vi "BasicDigitizerAcquire.vi"() -> ()   [LabVIEW 2014]
uses:
  Program Files (x86)/CAEN/Comm/labview/CAENComm.lvlib
panel:
  out "VernierTopHalves":i32[](array[numeric])
  out "QDC":u32[](array[numeric]) format="%.0x"
  in  "QDC module Base Address":u32 format="%.0x"
  in  "# of events before transfer":u16=1 min=1 max=32
  out "error out 2":errorcluster
  in  "# Rpts Vernier Cal":i32=100
  out "Min Ch0":u16
  out "max Ch0":u16
  out "Min Ch2":u16
  out "max Ch2":u16
  out "max Ch1":u16
  out "Min Ch1":u16
  out "Min Ch3":u16
  out "max Ch3":u16
  out "Verniers":u16[][](graph)
  out "End Idx":u16
  out "TRIG_REC":u8
  in  "MBLT?":bool
  out "Mean Time (secs)":dbl
  out "This Time (secs)":dbl
  out "RAW Wfm Plot":u16[](graph)
  in  "stop":bool
  in  "Software Trig?":bool
  in  "VME Base Address":u32=4026859520 format="%.0x"
  out "error out":errorcluster
  out "Wfm Plot":u16[][](graph)
  out "Ch1":u16[](array[numeric])
  out "Ch3":u16[](array[numeric])
  out "Ch0":u16[](array[numeric])
  out "Ch2":u16[](array[numeric])
  out "Channel Data (interleaved)":u32[](array[numeric])
  out "1st Sample, Verniers, and BL Reset":u16[](array[numeric])
  in  "# Samples after Trig":u16
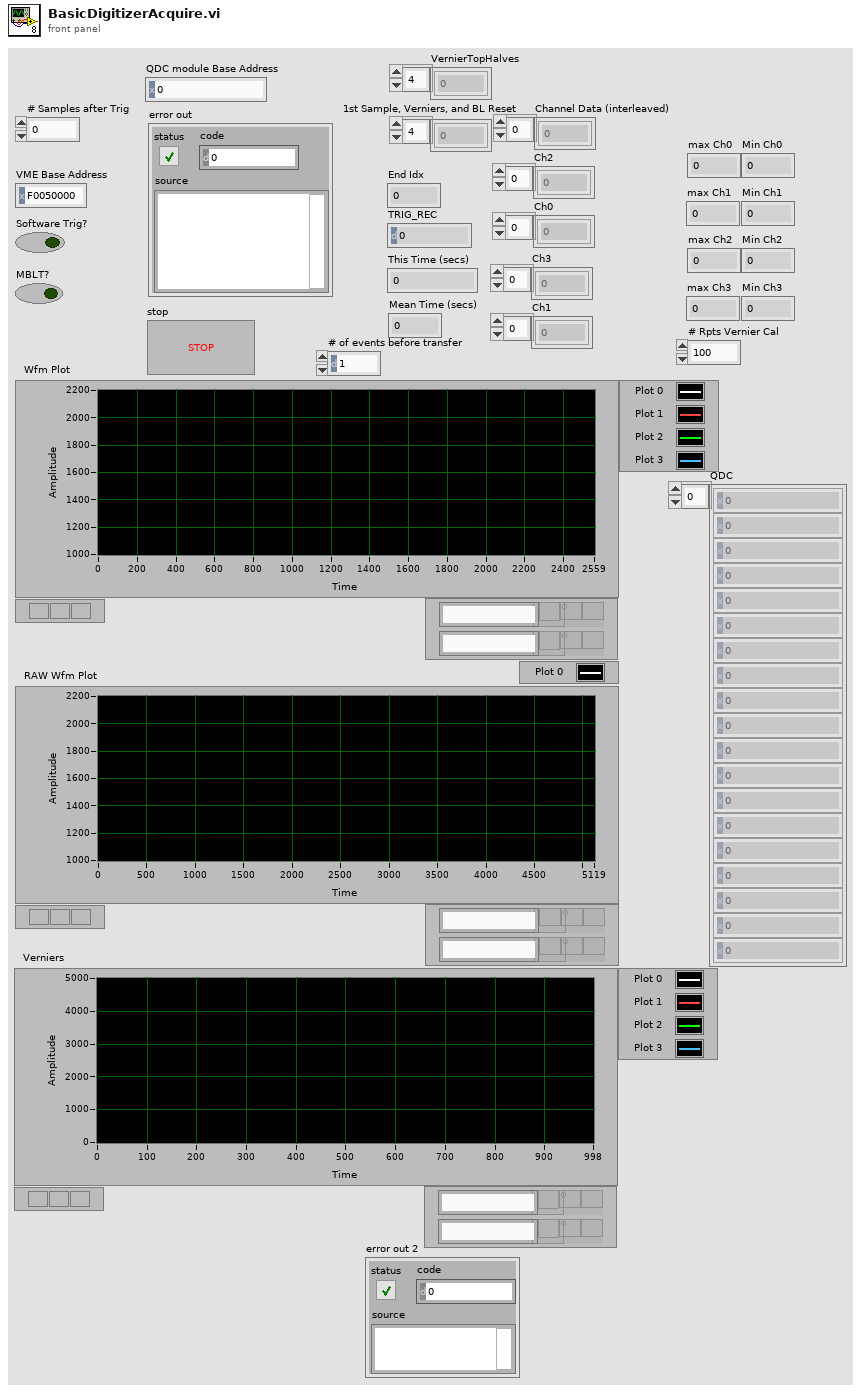
[diagram p1: front panel]
types:
  T1 = enum16{"Configure", "Initialise", "Run", "Close"}
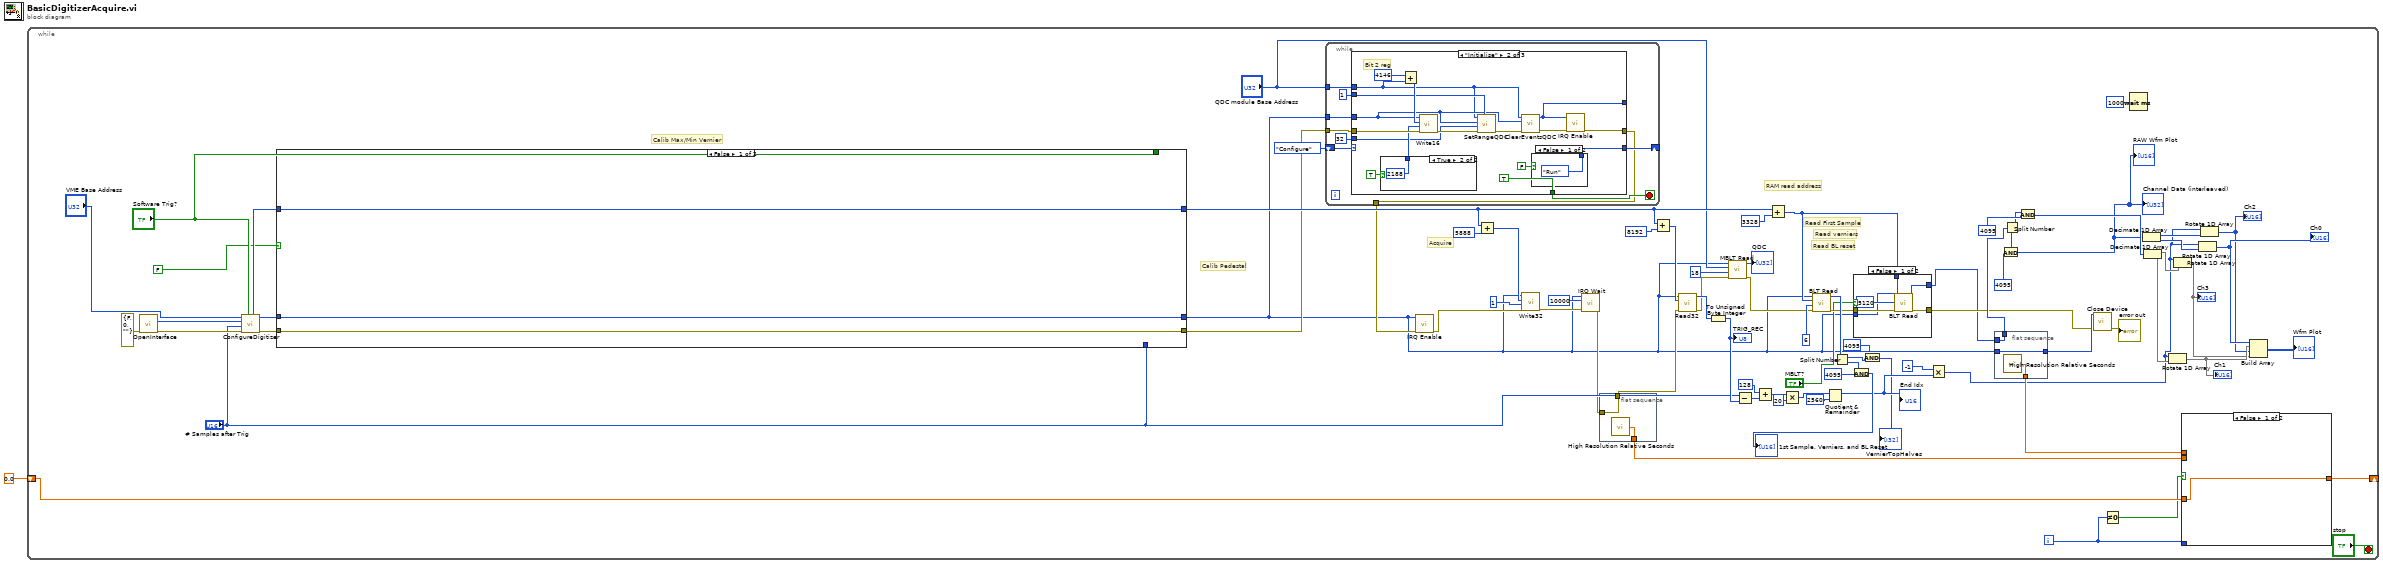
[diagram p0: block diagram]
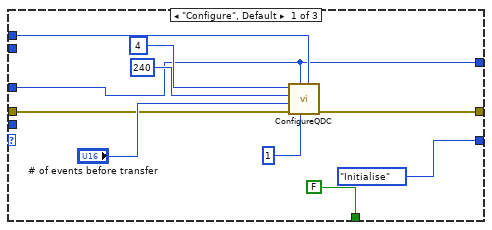
[diagram p2: hidden frame]
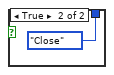
[diagram p3: hidden frame]
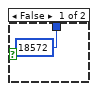
[diagram p4: hidden frame]
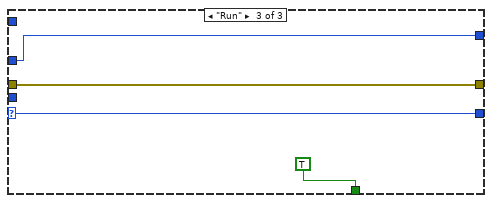
[diagram p5: hidden frame]
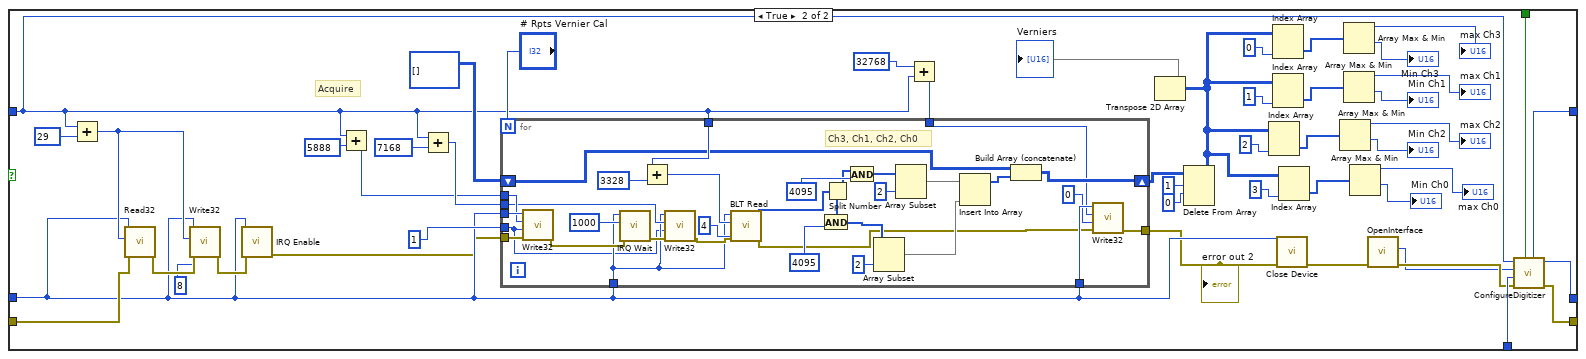
[diagram p6: hidden frame]
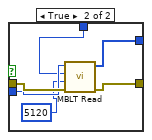
[diagram p7: hidden frame]
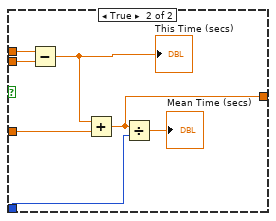
[diagram p8: hidden frame]
diagram:
  n1 = while {
    shift-right: [w56] -> _
    shift-left: 0.0 ("x-y") -> [w57]
    i -> [w55]
    stop <- "stop" stop-if-true
    # "Calib Max/Min Vernier"
    # "Read BL reset"
    # "Read verniers"
    # "Read First Sample"
    # "RAM read address"
    # "Acquire"
    # "Calib Pedestal"
    n2 = call "OpenInterface.vi"("error in (no error)"=errorcluster {"status"=FALSE, "code"=0, "source"=""}) -> ("error out"=w82:errorcluster, "handle"=w28:i32)  [unwired: 8 in, 1 out]
    n3 = call "ConfigureDigitizer.vi"("Software Trig?"="Software Trig?", "error in (no error)"=w82, "# Samples after Trig"="# Samples after Trig", "handle"=w28, "VME Base Address"="VME Base Address") -> ("error out"=w27:errorcluster, "handle out"=w20:i32, "VME Base Address out"=w24:u32)  [unwired: 4 in]
    n4 = case shown="False" FALSE ("Vernier Calib?") {
      tunnel: w27 -> [w128 w177]
      tunnel: [w128 w169] -> w12
      tunnel: "# Samples after Trig" -> [_ w168]
      tunnel: "Software Trig?" -> [_ w167]
      tunnel: w24 -> [w127 w132]
      tunnel: [w127 w166] -> w14
      tunnel: [w129 w165] -> w5
      tunnel: w20 -> [w129 w136]
      frame False {
      }
      frame True {
        # "Acquire"
        n5 = Add(x=w132, y=u32 29) -> (x+y=w174:u32)
        n6 = call "Read32.vi"("error in (no error)"=w177, "Address"=w174, "handle"=w136) -> ("error out"=w175:errorcluster)  [unwired: 7 in, 1 out]
        n7 = call "Write32.vi"("error in (no error)"=w175, "Data"=u32 8, "Address"=w174, "handle"=w136) -> ("error out"=w170:errorcluster)  [unwired: 7 in]
        n8 = call "IRQ Enable.vi"("error in (no error)"=w170, "handle"=w136) -> ("error out"=w130:errorcluster)  [unwired: 9 in]
        n9 = Add(x=w132, y=u32 5888 ("x")) -> (x+y=w131:u32)
        n10 = Add(x=w132, y=u32 7168 ("x")) -> (x+y=w138:u32)
        n11 = Add(x=u32 32768, y=w132) -> (x+y=w134:u32)
        n12 = for {
          N: "# Rpts Vernier Cal" -> [_]
          tunnel: w132 -> [w198]
          tunnel: w136 -> [w180]
          shift-right: [w194] -> w158
          shift-left: u16[][] [] -> [w193]
          tunnel: w136 -> [w191]
          tunnel: w138 -> [w181]
          tunnel: u32 1 ("Data") -> [w179]
          tunnel: w136 -> [w189]
          tunnel: w134 -> [w188]
          tunnel: [w186] -> w133
          tunnel: w131 -> [w183]
          tunnel: w130 -> [w182]
          # "Ch3, Ch1, Ch2, Ch0"
          n13 = call "Write32.vi"("error in (no error)"=w182, "Data"=w179, "Address"=w183, "handle"=w191) -> ("error out"=w192:errorcluster)  [unwired: 7 in]
          n14 = call "IRQ Wait.vi"("error in (no error)"=w192, "Timeout"=u32 1000, "handle"=w180) -> ("error out"=w185:errorcluster)  [unwired: 8 in]
          n15 = Add(x=w198, y=u32 3328 ("x")) -> (x+y=w190:u32)
          n16 = call "Write32.vi"("error in (no error)"=w185, "Data"=w179, "Address"=w181, "handle"=w180) -> ("error out"=w184:errorcluster)  [unwired: 7 in]
          n17 = call "BLT Read.vi"("error in (no error)"=w184, "BltSize"=4, "Address"=w190, "handle"=w180) -> ("error out"=w178:errorcluster, "Buff"=w203:u32[])  [unwired: 5 in, 1 out]
          n18 = Split Number(x=w203) -> (hi(x)=w204:u16[], lo(x)=w207:u16[])
          n19 = And(x=w207, y=u16 4095 ("Numeric")) -> (x .and. y?=w199:u16[])
          n20 = And(x=w204, y=u16 4095 ("Numeric")) -> (x .and. y?=w202:u16[])
          n21 = Array Subset(array=w199, index=2) -> (w196:u16[])  [unwired: 1 in]
          n22 = Array Subset(array=w202, index=2) -> (w197:u16[])  [unwired: 1 in]
          n23 = Insert Into Array(array=w197, new element=w196) -> (w195:u16[])  [unwired: 1 in]
          n24 = Build Array (concatenate)(w193, w195) -> (w194:u16[][])
          n25 = call "Write32.vi"("error in (no error)"=w178, "Data"=u32 0, "Address"=w188, "handle"=w189) -> ("error out"=w186:errorcluster)  [unwired: 7 in]
        }
        "error out 2" <- w133
        n26 = Delete From Array(array=w158, length=1, index (row)=0) -> (array with subset deleted=w147:u16[][])  [unwired: 1 in, 1 out]
        n27 = Transpose 2D Array(2D array=w147) -> (transposed array=→"Verniers":u16[][])
        n28 = Index Array(array=w147, index (col)=2 ("index (row)")) -> (element=w151:u16[])  [unwired: 1 in]
        n29 = Index Array(array=w147, index (col)=0 ("index (row)")) -> (element=w157:u16[])  [unwired: 1 in]
        n30 = Index Array(array=w147, index (col)=1 ("index (row)")) -> (element=w152:u16[])  [unwired: 1 in]
        n31 = call "Close Device.vi"("error in (no error)"=w133, "handle"=w136) -> ("error out"=w162:errorcluster)  [unwired: 9 in]
        n32 = Index Array(array=w147, index (col)=3 ("index (row)")) -> (element=w148:u16[])  [unwired: 1 in]
        n33 = Array Max & Min(array=w151) -> (max value=→"max Ch2":u16, min value=→"Min Ch2":u16)  [unwired: 2 out]
        n34 = Array Max & Min(array=w157) -> (max value=→"max Ch3":u16, min value=→"Min Ch3":u16)  [unwired: 2 out]
        n35 = Array Max & Min(array=w152) -> (max value=→"max Ch1":u16, min value=→"Min Ch1":u16)  [unwired: 2 out]
        n36 = Array Max & Min(array=w148) -> (max value=→"max Ch0":u16, min value=→"Min Ch0":u16)  [unwired: 2 out]
        n37 = call "OpenInterface.vi"("error in (no error)"=w162) -> ("error out"=w161:errorcluster, "handle"=w160:i32)  [unwired: 8 in, 1 out]
        n38 = call "ConfigureDigitizer.vi"("Software Trig?"=w167, "error in (no error)"=w161, "# Samples after Trig"=w168, "handle"=w160, "VME Base Address"=w132) -> ("error out"=w169:errorcluster, "handle out"=w165:i32, "VME Base Address out"=w166:u32)  [unwired: 4 in]
      }
    }
    n39 = while {
      tunnel: "QDC module Base Address" -> [w91]
      tunnel: w5 -> [w88]
      tunnel: w12 -> [w87]
      shift-right: [w85] -> _
      shift-left: T1."Configure" -> [w83]
      tunnel: [w84] -> w11
      stop <- w86 stop-if-true
      n40 = case shown="\"Initialise\"" w83 {
        selector: w83 -> [_ _ w126]
        tunnel: [w97 w102 w125] -> w84
        tunnel: [w93 w106 w124] -> _
        tunnel: w87 -> [w92 w118 w125]
        tunnel: w91 -> [w96 w109 _]
        tunnel: w88 -> [w93 w110 w124]
        tunnel: u16 32 ("High range threshold") -> [_ w113 _]
        tunnel: u16 1 ("handle out") -> [_ w112 _]
        tunnel: [T1."Initialise" w108 w126] -> w85
        tunnel: [FALSE TRUE TRUE] -> w86
        frame "Configure", Default {
          n41 = call "ConfigureQDC.vi"("VME module Base Address"=w96, "IRQ Lvl"=u16 1, "handle"=w93, "error in (no error)"=w92, "# of events before transfer (max 32)"="# of events before transfer", "CBLT Addr"=u16 240, "Geo Addr"=u16 4) -> ("error out"=w97:errorcluster)  [unwired: 4 in]
        }
        frame "Initialise" {
          # "Bit 2 reg"
          n42 = case shown="True" TRUE {
            tunnel: [18572 2188] -> w115
            frame False {
            }
            frame True {
            }
          }
          n43 = Add(x=u32 4146, y=w109) -> (x+y=w116:u32)
          n44 = call "Write16.vi"("error in (no error)"=w118, "Data"=w115, "Address"=w116, "handle"=w110) -> ("error out"=w114:errorcluster)  [unwired: 7 in]
          n45 = call "SetRangeQDC.vi"("Low Range threshold"=w112, "error in (no error)"=w114, "High range threshold"=w113, "handle"=w110, "VME module Base Address"=w109) -> ("error out"=w111:errorcluster)  [unwired: 6 in]
          n46 = call "ClearEventsQDC.vi"("error in (no error)"=w111, "handle"=w110, "VME module Base Address"=w109) -> ("error out"=w107:errorcluster, "handle out"=w106:i32)  [unwired: 6 in, 1 out]
          n47 = case shown="False" FALSE {
            tunnel: [T1."Run" T1."Close"] -> w108
            frame False {
            }
            frame True {
            }
          }
          n48 = call "IRQ Enable.vi"("error in (no error)"=w107, "handle"=w106) -> ("error out"=w102:errorcluster)  [unwired: 9 in]
        }
        frame "Run" {
        }
      }
    }
    n49 = call "IRQ Enable.vi"("error in (no error)"=w11, "handle"=w5) -> ("error out"=w17:errorcluster)  [unwired: 9 in]
    n50 = Add(x=w14, y=u32 5888 ("x")) -> (x+y=w71:u32)
    n51 = call "Write32.vi"("error in (no error)"=w17, "Data"=u32 1, "Address"=w71, "handle"=w5) -> ("error out"=w73:errorcluster)  [unwired: 7 in]
    n52 = call "IRQ Wait.vi"("error in (no error)"=w73, "Timeout"=u32 10000, "handle"=w5) -> ("error out"=w16:errorcluster)  [unwired: 8 in]
    n53 = flat-sequence {
      tunnel: [w232] -> w67
      tunnel: w16 -> [w231]
      tunnel: [w231] -> w15
      frame #0 {
        n54 = call <vilib>:"High Resolution Relative Seconds.vi"() -> ("relative seconds"=w232:dbl)
      }
    }
    n55 = Add(x=w14, y=u32 8192 ("x")) -> (x+y=w46:u32)
    n56 = call "Read32.vi"("error in (no error)"=w15, "Address"=w46, "handle"=w5) -> ("error out"=w10:errorcluster, "Data"=w45:u32)  [unwired: 7 in]
    n57 = To Unsigned Byte Integer(number=w45) -> (unsigned 8bit integer=w44:u8)
    "TRIG_REC" <- w44
    n58 = call "MBLT Read.vi"("error in (no error)"=w10, "BltSize"=18, "Address"="QDC module Base Address", "handle"=w5) -> ("error out"=w9:errorcluster, "Buff"=→"QDC":u32[])  [unwired: 5 in, 1 out]
    n59 = Subtract(x="# Samples after Trig", y=w44) -> (x-y=w43:u16)
    n60 = Add(x=u16 128, y=w43) -> (x+y=w41:u16)
    n61 = Add(x=w14, y=u32 3328 ("x")) -> (x+y=w80:u32)
    n62 = Multiply(x=w41, y=u16 20) -> (x*y=w39:u16)
    n63 = call "BLT Read.vi"("error in (no error)"=w9, "BltSize"=6, "Address"=w80, "handle"=w5) -> ("error out"=w51:errorcluster, "Buff"=w66:u32[])  [unwired: 5 in, 1 out]
    n64 = Quotient & Remainder(x=w39, y=u16 2560) -> (x-y*floor(x/y)=w32:u16)  [unwired: 1 out]
    "End Idx" <- w32
    n65 = Split Number(x=w66) -> (hi(x)=w4:u16[], lo(x)=w65:u16[])
    n66 = And(x=w65, y=4095 ("Numeric")) -> (x .and. y?=→"1st Sample, Verniers, and BL Reset":i32[])
    n67 = case shown="False" "MBLT?" {
      tunnel: w80 -> [w216 w218]
      tunnel: [w214 w221] -> w48
      tunnel: w51 -> [w213 w222]
      tunnel: [w212 w220] -> w49
      tunnel: w5 -> [w211 w219]
      frame False {
        n68 = call "BLT Read.vi"("error in (no error)"=w213, "BltSize"=5120, "Address"=w216, "handle"=w211) -> ("error out"=w212:errorcluster, "Buff"=w214:u32[])  [unwired: 5 in, 1 out]
      }
      frame True {
        n69 = call "MBLT Read.vi"("error in (no error)"=w222, "BltSize"=5120, "Address"=w218, "handle"=w219) -> ("error out"=w220:errorcluster, "Buff"=w221:u32[])  [unwired: 5 in, 1 out]
      }
    }
    n70 = And(x=4095 ("Numeric"), y=w4) -> (x .and. y?=→"VernierTopHalves":i32[])
    n71 = Multiply(x=i16 -1, y=w32) -> (x*y=w30:u16)
    n72 = flat-sequence {
      tunnel: [w235] -> w69
      tunnel: w5 -> [w235]
      tunnel: [w234] -> w68
      tunnel: w48 -> [w233]
      tunnel: [w233] -> w52
      frame #0 {
        n73 = call <vilib>:"High Resolution Relative Seconds.vi"() -> ("relative seconds"=w234:dbl)
      }
    }
    n74 = Split Number(x=w52) -> (hi(x)=w59:u16[], lo(x)=w62:u16[])
    n75 = And(x=w62, y=u16 4095 ("Numeric")) -> (x .and. y?=w53:u16[])
    "Channel Data (interleaved)" <- w53
    "RAW Wfm Plot" <- w53
    n76 = And(x=w59, y=u16 4095 ("Numeric")) -> (x .and. y?=w58:u16[])
    n77 = call "Close Device.vi"("error in (no error)"=w49, "handle"=w69) -> ("error out"=→"error out":errorcluster)  [unwired: 9 in]
    n78 = Not Equal To 0?(x=w55) -> (x != 0?=w54:bool)
    n79 = Wait (ms)(milliseconds to wait=u32 1000) -> ()  [unwired: 1 out]
    n80 = Decimate 1D Array(w53) -> (w37:u16[], w36:u16[])
    n81 = Decimate 1D Array(w58) -> (w34:u16[], w33:u16[])
    n82 = Rotate 1D Array(1:w33, 2:w30) -> (0:w23:u16[])
    "Ch1" <- w23
    n83 = Rotate 1D Array(1:w34, 2:w30) -> (0:w22:u16[])
    "Ch3" <- w22
    n84 = case shown="False" w54 {
      tunnel: w68 -> [_ w230]
      tunnel: w67 -> [_ w229]
      tunnel: w57 -> [w223 w227]
      tunnel: w55 -> [_ w226]
      tunnel: [w223 w224] -> w56
      frame False {
      }
      frame True {
        n85 = Subtract(x=w230, y=w229) -> (x-y=w228:dbl)
        "This Time (secs)" <- w228
        n86 = Add(x=w228, y=w227) -> (x+y=w224:dbl)
        n87 = Divide(x=w224, y=w226) -> (x/y=→"Mean Time (secs)":dbl)
      }
    }
    n88 = Rotate 1D Array(1:w36, 2:w30) -> (0:w35:u16[])
    "Ch0" <- w35
    n89 = Rotate 1D Array(1:w37, 2:w30) -> (0:w21:u16[])
    "Ch2" <- w21
    n90 = Build Array(w35, w23, w21, w22) -> (→"Wfm Plot":u16[][])
  }
